vi "Polarization check.vi"() -> ()   [LabVIEW 2014]
uses:
  <vilib>/Analysis/baseanly.llb/Mean (DBL).vi
  Main-Stage-Based/(Global) Current handle and LaserPower_YCC.vi
  <vilib>/Analysis/NI_AALBase.lvlib
  <vilib>/gmath/NI_Gmath.lvlib
  <vilib>/Analysis/NI_AALPro.lvlib
panel:
  in  "record time (s)":dbl=0.5
  out "correlation coefficient r":dbl format="%.7g"
  out "ky (pN/nm)":dbl
  in  "y-Convf-cal-array":dbl[](array[numeric])=[0.063191, -0.059867]
  in  "x-Convf-cal-array":dbl[](array[numeric])=[0.10341, -0.29934]
  out "kx (pN/nm)":dbl
  in  "Temp (C)":dbl=24.0
  out "r^2":dbl format="%.7g"
  out "STDy (nm)":dbl format="%0.2f"
  out "STDx (nm)":dbl format="%0.2f"
  out "XY Graph":cluster{dbl[], "Best Linear Fit":dbl[]}[](graph)
  out "y position (nm)":dbl[](array[numeric])
  out "x position (nm)":dbl[](array[numeric])
  out "y position (V)":dbl[](array[numeric])
  out "x position (V)":dbl[](array[numeric])
  in  "rate":dbl=32000.0
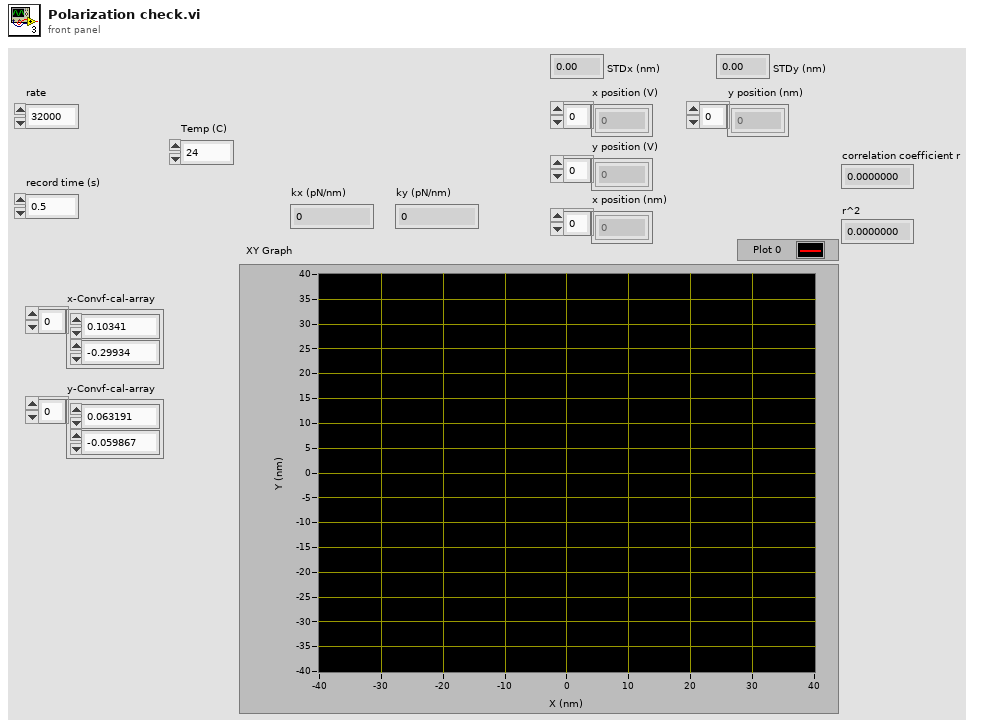
[diagram p1: front panel]
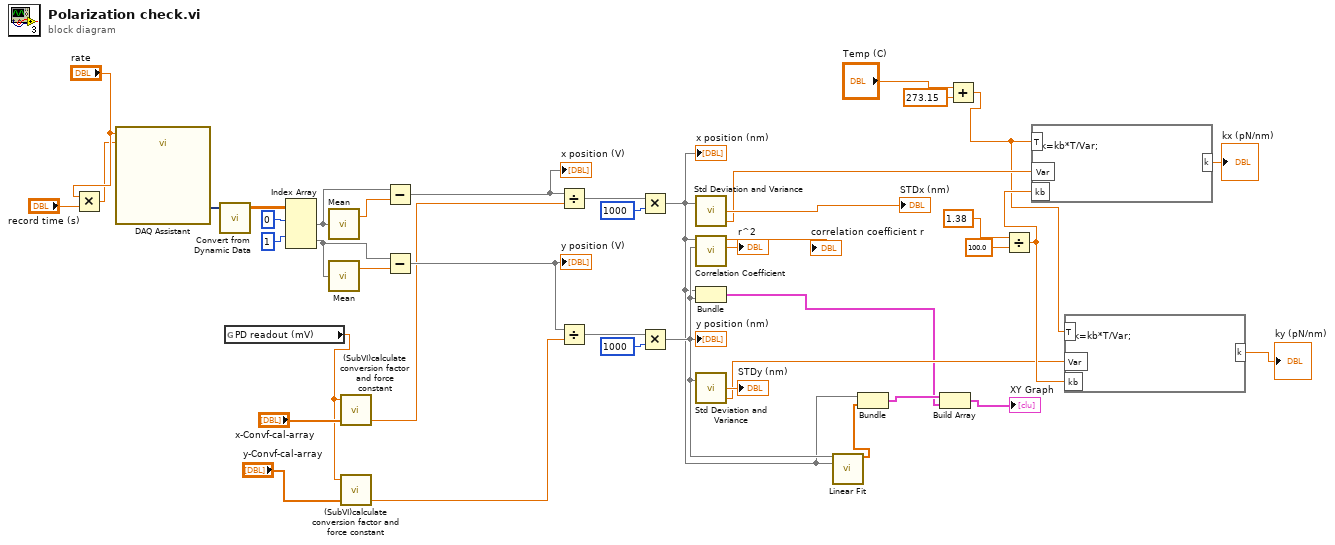
[diagram p0: block diagram]
diagram:
  n1 = Multiply(x="rate", y="record time (s)") -> (x*y=w7:dbl)
  n2 = call "DAQ Assistant"("rate"="rate", "number of samples"=w7) -> ("data"=w42:dynamicdata)  [unwired: 15 in, 2 out]
  n3 = call "Convert from Dynamic Data"("Dynamic Data Type"=w42) -> ("Array"=w41:dbl[][])  [unwired: 3 in]
  n4 = global read "(Global) Current handle and LaserPower_YCC.vi" "PD readout (mV)"() -> (w17:dbl)
  n5 = Index Array(array=w41, index (row) #1=0 ("index (row)"), index (row) #2=1 ("index (row)")) -> (element #1=w38:dbl[], element #2=w35:dbl[])  [unwired: 2 in]
  n6 = call-poly <vilib>:"Mean.vi"("X"=w38) -> ("mean"=w37:dbl)  [unwired: 1 out]
  n7 = call-poly <vilib>:"Mean.vi"("X"=w35) -> ("mean"=w36:dbl)  [unwired: 1 out]
  n8 = call "(SubVI)calculate conversion factor and force constant.vi"("Convf-cal-array"="x-Convf-cal-array", "laser power (mW)"=w17) -> ("conversion factor (V/um)"=w16:dbl)  [unwired: 2 in, 1 out]
  n9 = call "(SubVI)calculate conversion factor and force constant.vi"("Convf-cal-array"="y-Convf-cal-array", "laser power (mW)"=w17) -> ("conversion factor (V/um)"=w15:dbl)  [unwired: 2 in, 1 out]
  n10 = Subtract(x=w38, y=w37) -> (x-y=w34:dbl[])
  "x position (V)" <- w34
  n11 = Subtract(x=w35, y=w36) -> (x-y=w33:dbl[])
  "y position (V)" <- w33
  n12 = Divide(x=w34, y=w16) -> (x/y=w32:dbl[])
  n13 = Divide(x=w33, y=w15) -> (x/y=w29:dbl[])
  n14 = Multiply(x=w32, y=1000) -> (x*y=w5:dbl[])
  "x position (nm)" <- w5
  n15 = Multiply(x=w29, y=1000) -> (x*y=w6:dbl[])
  "y position (nm)" <- w6
  n16 = call <vilib>:"Std Deviation and Variance.vi"("X"=w5) -> ("standard deviation"=→"STDx (nm)":dbl, "variance"=w23:dbl)  [unwired: 1 in, 1 out]
  n17 = call <vilib>:"Correlation Coefficient.vi"("Y"=w6, "X"=w5) -> ("r^2"=→"r^2":dbl, "correlation coefficient r"=→"correlation coefficient r":dbl)  [unwired: 8 in]
  n18 = Bundle(w5, w6) -> (w2:cluster{dbl[], dbl[]})  [unwired: 1 in]
  n19 = call <vilib>:"Std Deviation and Variance.vi"("X"=w6) -> ("standard deviation"=→"STDy (nm)":dbl, "variance"=w12:dbl)  [unwired: 1 in, 1 out]
  n20 = call <vilib>:"Linear Fit.vi"("Y"=w6, "X"=w5) -> ("Best Linear Fit"=w4:dbl[])  [unwired: 9 in, 4 out]
  n21 = Bundle(w5, "Best Linear Fit"=w4) -> (w3:cluster{dbl[], "Best Linear Fit":dbl[]})  [unwired: 1 in]
  n22 = Build Array(w3, w2) -> (→"XY Graph":cluster{dbl[], "Best Linear Fit":dbl[]}[])
  n23 = Add(x="Temp (C)", y=273.15) -> (x+y=w13:dbl)
  n24 = Divide(x=1.38 ("input variable"), y=100.0) -> (x/y=w14:dbl)
  n25 = formula code=";\nk=kb*T/Var;"("T"=w13, "Var"=w23, "kb"=w14) -> ("k"=→"kx (pN/nm)":dbl)
  n26 = formula code=";\nk=kb*T/Var;"("T"=w13, "Var"=w12, "kb"=w14) -> ("k"=→"ky (pN/nm)":dbl)
